vi "Disconnected.vi"(8 "error in (no error)":errorcluster, 11 "Arduino_TranslationStage_UI.lvlib:Arduino_Stepper.lvclass":refnum<class "Arduino_Stepper.lvclass">) -> (0 "error out":errorcluster, 3 "Arduino_TranslationStage_UI.lvlib:Arduino_Stepper.lvclass":refnum<class "Arduino_Stepper.lvclass">)   [LabVIEW 2023, in "Arduino_TranslationStage_UI.lvlib" / "Arduino_Stepper.lvclass"]
uses:
  Arduino_Stepper.lvclass
  Arduino_Stepper.lvclass/Arduino_Stepper.ctl
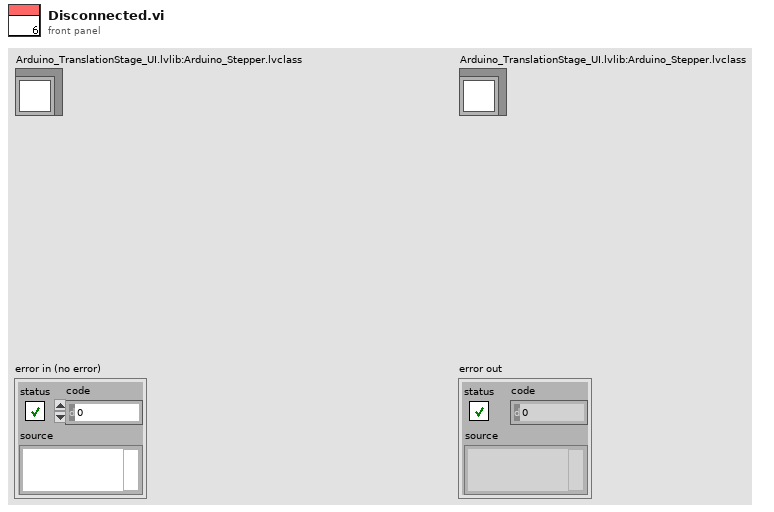
[diagram p1: front panel]
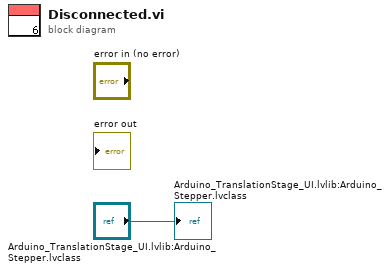
[diagram p0: block diagram]
diagram:
  "Arduino_TranslationStage_UI.lvlib:Arduino_Stepper.lvclass" <- "Arduino_TranslationStage_UI.lvlib:Arduino_Stepper.lvclass"
